vi "syncDAQ.vi"() -> ()   [LabVIEW 2013]
uses:
  <vilib>/Utility/error.llb/DialogType.ctl
  <vilib>/DAQmx/read.llb/DAQmx Read (Analog 1D Wfm NChan NSamp).vi
  <vilib>/DAQmx/miscellaneous.llb/DAQmx Fill In Error Info.vi
  <vilib>/ErrorRing/Error Ring.xnode
panel:
  in  "Ratio":dbl=0.2 caption="复位时间比"
  in  "Vx_Max":dbl=3.0 caption="X向最大电压"
  in  "Vy_Max":dbl=3.0 caption="Y向最大电压"
  in  "N_x":i32=512 caption="采样行数"
  in  "N_y":i32=512 caption="每行采样数"
  in  "sample mode":i32(ring)=1 caption="采样模式" items=["有限采样", "连续采样", "硬件定时单点"]
  in  "停止按钮":bool
  in  "每次采集行数":i32=32
  in  "physical channels read":tag="Dev1/ai0" caption="物理通道（读取）"
  in  "physical channels write":tag="Dev1/ao0:1" caption="物理通道（写入）"
  out "number of samples\nper channel":i32=16384 caption="每通道采样数"
  in  "timing source":tag="OnboardClock" caption="定时源"
  in  "rate":dbl=1000000.0 caption="采样速率" format="%#_6f"
  out "data read 2":waveform(dbl)[](graph) caption="数据输出"
  out "data read":waveform(dbl)[](graph) caption="数据输出"
  out "data write":waveform(dbl)[](graph) caption="数据输出"
  # "Basic DAQ\nsettings"
  # "Imaging settings"
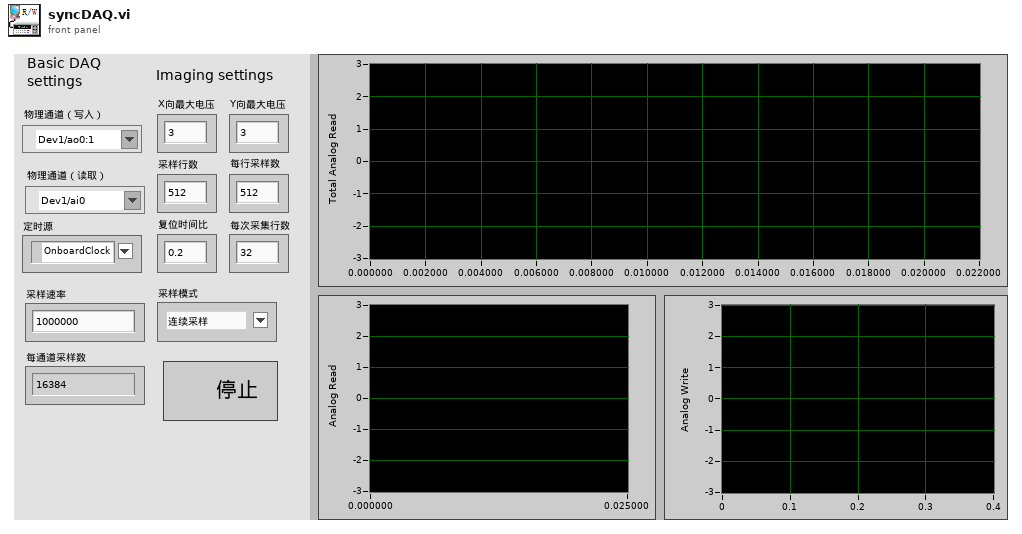
[diagram p1: front panel]
types:
  T1 = typedef "DialogType.ctl" = u16
  T2 = cluster{"Vx_Max":dbl, "Vy_Max":dbl, "Tx":dbl, "Row_N":i32, "Ratio":dbl}
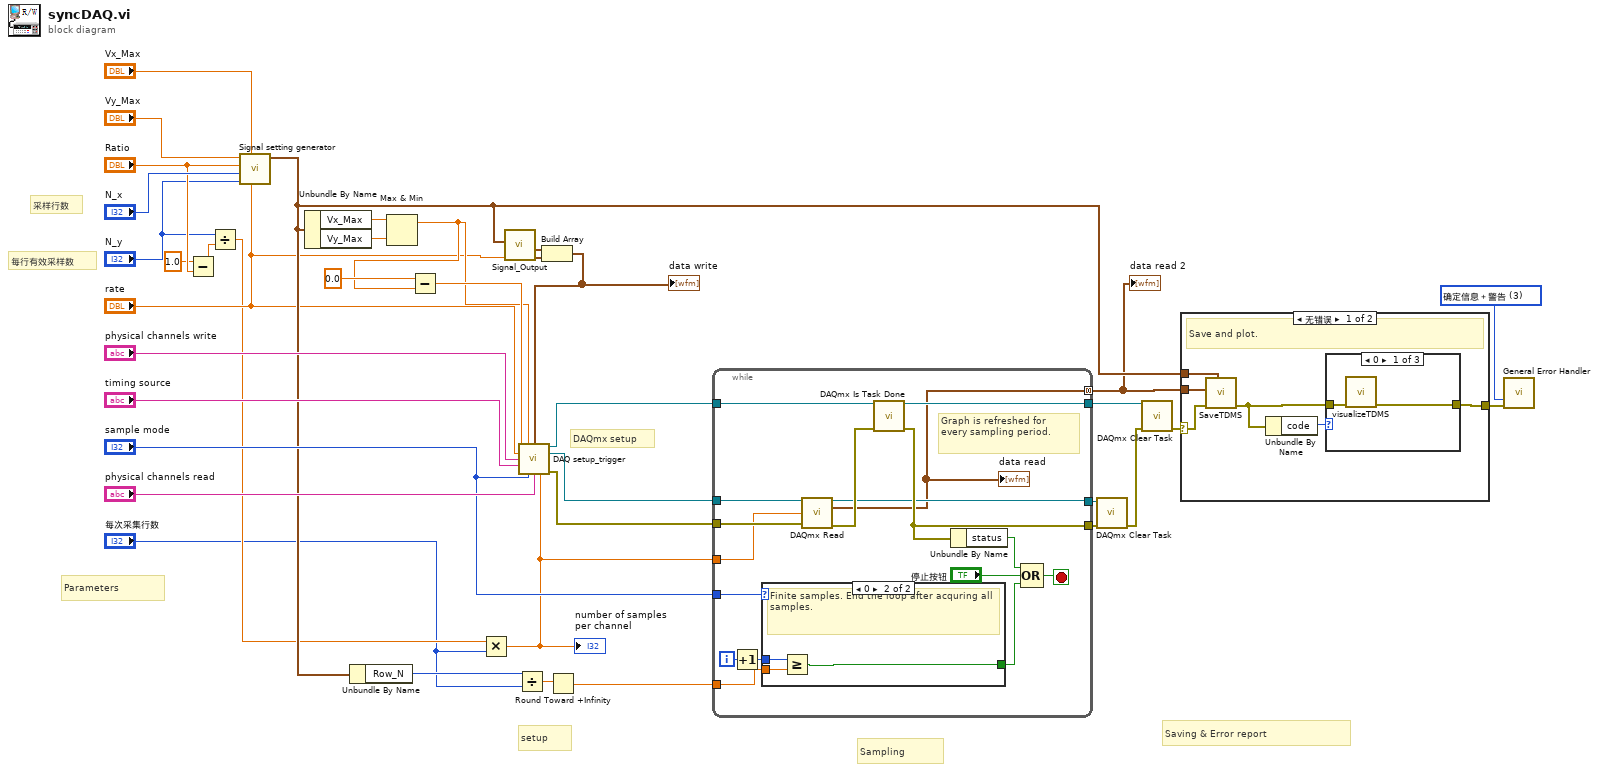
[diagram p0: block diagram]
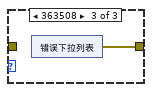
[diagram p3: hidden frame]
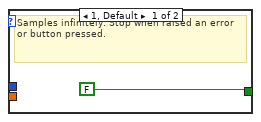
[diagram p5: hidden frame]
diagram:
  w33 = T1 3 items=["无对话框", "确定信息", "继续或停止信息", "确定信息＋警告", "继续/停止+警告"] ("type of dialog (OK msg:1)")
  # "每行有效采样数"
  # "采样行数"
  # "DAQmx setup"
  # "Parameters"
  # "Saving & Error report"
  # "Sampling"
  # "setup"
  n1 = Subtract(x=1.0, y="Ratio") -> (x-y=w8:dbl)
  n2 = Divide(x="N_y", y=w8) -> (x/y=w7:dbl)
  n3 = call "Signal setting generator.vi"("rate"="rate", "Vx_Max"="Vx_Max", "N_y"="N_y", "N_x"="N_x", "Ratio"="Ratio", "Vy_Max"="Vy_Max") -> ("Waveform out"=w17:T2)  [unwired: 5 in]
  n4 = Unbundle By Name(w17) -> ("Vx_Max"=w20:dbl, "Vy_Max"=w19:dbl)
  n5 = Unbundle By Name(w17) -> ("Row_N"=w4:i32)
  n6 = Max & Min(x=w20, y=w19) -> (max(x,y)=w18:dbl)  [unwired: 1 out]
  n7 = Subtract(x=0.0, y=w18) -> (x-y=w28:dbl)
  n8 = Multiply(x=w7, y="每次采集行数") -> (x*y=w12:dbl)
  "number of samples\nper channel" <- w12
  n9 = call "Signal_Output.vi"("Fs (Hz)"="rate", "Waveform settings"=w17) -> ("Y"=w22:waveform(dbl), "X"=w23:waveform(dbl))  [unwired: 7 in, 1 out]
  n10 = Divide(x=w4, y="每次采集行数") -> (x/y=w2:dbl)
  n11 = Build Array(w23, w22) -> (w6:waveform(dbl)[])
  "data write" <- w6
  n12 = call "DAQ setup_trigger.vi"("Vx_min"=w28, "Vx_max"=w18, "数组"=w6, "rate"="rate", "physical channels write"="physical channels write", "Timing source"="timing source", "sample mode"="sample mode", "physical channels read"="physical channels read", "Number of samples per channel"=w12) -> ("Writing task out"=w38:refnum<k21>, "Reading task out"=w32:refnum<k21>, "错误输出"=w31:errorcluster)  [unwired: 4 in]
  n13 = Round Toward +Infinity(x=w2) -> (ceil(x): smallest int >= x=w1:dbl)
  n14 = while {
    tunnel: w32 -> [w49]
    tunnel: w38 -> [w52]
    tunnel: w31 -> [w50]
    tunnel: [w54] -> w36
    tunnel: [w53] -> w37
    tunnel: [w51] -> w35
    tunnel: w12 -> [w48]
    tunnel: w1 -> [w47]
    tunnel: "sample mode" -> [w42]
    tunnel: [w41] -> w5 mode=concatenating
    i -> [w40]
    stop <- w46 stop-if-true
    # "Graph is refreshed for\nevery sampling period."
    n15 = Increment(x=w40) -> (x+1=w39:i32)
    n16 = case "条件结构" shown="0" w42 {
      tunnel: w39 -> [_ w59]
      tunnel: w47 -> [_ w58]
      tunnel: [FALSE w57] -> w43
      frame 1, Default {
        # "Samples infinitely. Stop when raised an error or button pressed."
      }
      frame 0 {
        # "Finite samples. End the loop after acquring all samples."
        n17 = Greater Or Equal?(x=w59, y=w58) -> (x >= y?=w57:bool)
      }
    }
    n18 = call-poly <vilib>:"DAQmx Read.vi"("task/channels in"=w49, "number of samples per channel"=w48, "error in"=w50) -> ("task out"=w53:refnum<k21>, "data"=w41:waveform(dbl)[], "error out"=w55:errorcluster)  [unwired: 10 in]
    "data read" <- w41
    n19 = call <vilib>:"DAQmx Is Task Done.vi"("task/channels in"=w52, "error in"=w55) -> ("task out"=w51:refnum<k21>, "error out"=w54:errorcluster)  [unwired: 11 in, 1 out]
    n20 = Unbundle By Name(w54) -> ("status"=w45:bool)
    n21 = Compound Arithmetic op=OR(w45, "停止按钮", w43) -> (w46:bool)
  }
  "data read 2" <- w5
  n22 = call <vilib>:"DAQmx Clear Task.vi"("task in"=w37, "error in"=w36) -> ("error out"=w34:errorcluster)  [unwired: 13 in]
  n23 = call <vilib>:"DAQmx Clear Task.vi"("task in"=w35, "error in"=w34) -> ("error out"=w21:errorcluster)  [unwired: 13 in]
  n24 = case "条件结构" shown="无错误" w21 {
    selector: w21 -> [w64 w71]
    tunnel: w5 -> [w65 _]
    tunnel: [w61 w71] -> w24
    tunnel: w17 -> [w60 _]
    frame No Error {
      # "Save and plot."
      n25 = call "SaveTDMS.vi"("Waveform settings"=w60, "错误输入（无错误）"=w64, "数据"=w65) -> ("错误输出"=w63:errorcluster)  [unwired: 8 in]
      n26 = Unbundle By Name(w63) -> ("code"=w62:i32)
      n27 = case shown="0" w62 {
        tunnel: w63 -> [w67 w68 _]
        tunnel: [w66 w68 w69] -> w61
        frame 0 {
          n28 = call "visualizeTDMS.vi"("错误输入（无错误）"=w67) -> ("错误输出"=w66:errorcluster)  [unwired: 8 in, 2 out]
        }
        frame Default {
        }
        frame 363508 {
          n29 = xnode "错误下拉列表"() -> ("错误输出"=w69:errorcluster)
        }
      }
    }
    frame Error {
    }
  }
  n30 = call <vilib>:"General Error Handler.vi"("type of dialog (OK msg:1)"=w33, "error in (no error)"=w24) -> ()  [unwired: 9 in, 5 out]
